vi "Mix Columns5.vi"(11 "State In":u16[][](array[numeric])) -> (3 "数组":u16[][](array[numeric]))   [LabVIEW 2016, in "数据传输系统-04.lvlib"]
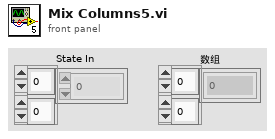
[diagram p1: front panel]
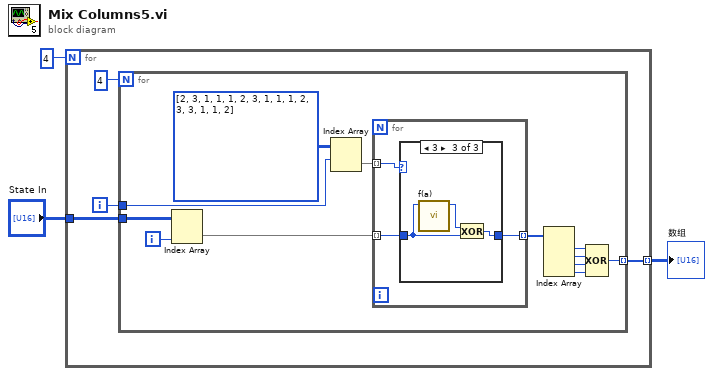
[diagram p0: block diagram]
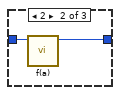
[diagram p3: hidden frame]
diagram:
  n1 = for {
    N: 4 -> [_]
    tunnel: "State In" -> [w7]
    tunnel: [w4] -> w2 mode=indexing
    i -> [w5]
    n2 = for {
      N: 4 -> [_]
      tunnel: w7 -> [w19]
      tunnel: w5 -> [w8]
      tunnel: [w10] -> w4 mode=indexing
      i -> [w9]
      n3 = Index Array(array=w19, index (col)=w9) -> (element=w17:u16[])  [unwired: 1 in]
      n4 = Index Array(array=i32[][] [[2, 3, 1, 1], [1, 2, 3, 1], [1, 1, 2, 3], [3, 1, 1, 2]] ("t[c]"), index (row)=w8) -> (element=w16:i32[])  [unwired: 1 in]
      n5 = for {
        tunnel: w17 -> [w22] mode=indexing
        tunnel: w16 -> [w21] mode=indexing
        tunnel: [w20] -> w15 mode=indexing
        n6 = case shown="3" w21 {
          tunnel: w22 -> [w23 w25 w27]
          tunnel: [w23 w24 w26] -> w20
          frame 1, Default {
          }
          frame 2 {
            n7 = call "f(a).vi"("x"=w25) -> ("数值"=w24:u16)  [unwired: 10 in]
          }
          frame 3 {
            n8 = call "f(a).vi"("x"=w27) -> ("数值"=w28:u16)  [unwired: 10 in]
            n9 = Exclusive Or(1:w27, 2:w28) -> (0:w26:u16)
          }
        }
      }
      n10 = Index Array(array=w15) -> (element #1=w14:u16, element #2=w13:u16, element #3=w12:u16, element #4=w11:u16)  [unwired: 4 in]
      n11 = Compound Arithmetic op=XOR(w14, w13, w12, w11) -> (w10:u16)
    }
  }
  "数组" <- w2
